vi "HW_QX - Parse Module Channel Parameters.vi"(8 "error in":errorcluster, 10 "sysModCFG[]":T5[](array[typedef]), 11 "AllDevRef[]":T3(array[cluster])) -> (0 "error out":errorcluster, 2 "InUsedDevRef[]":T3(array[cluster]), 3 "InUsedChan[]":T2)   [LabVIEW 2016]
uses:
  Ctrls/HardWare _ Channel Parameters.ctl
  Ctrls/HardWare _ Module Configuration.ctl
panel:
  out "AllModuPara[]":T4(array[cluster])
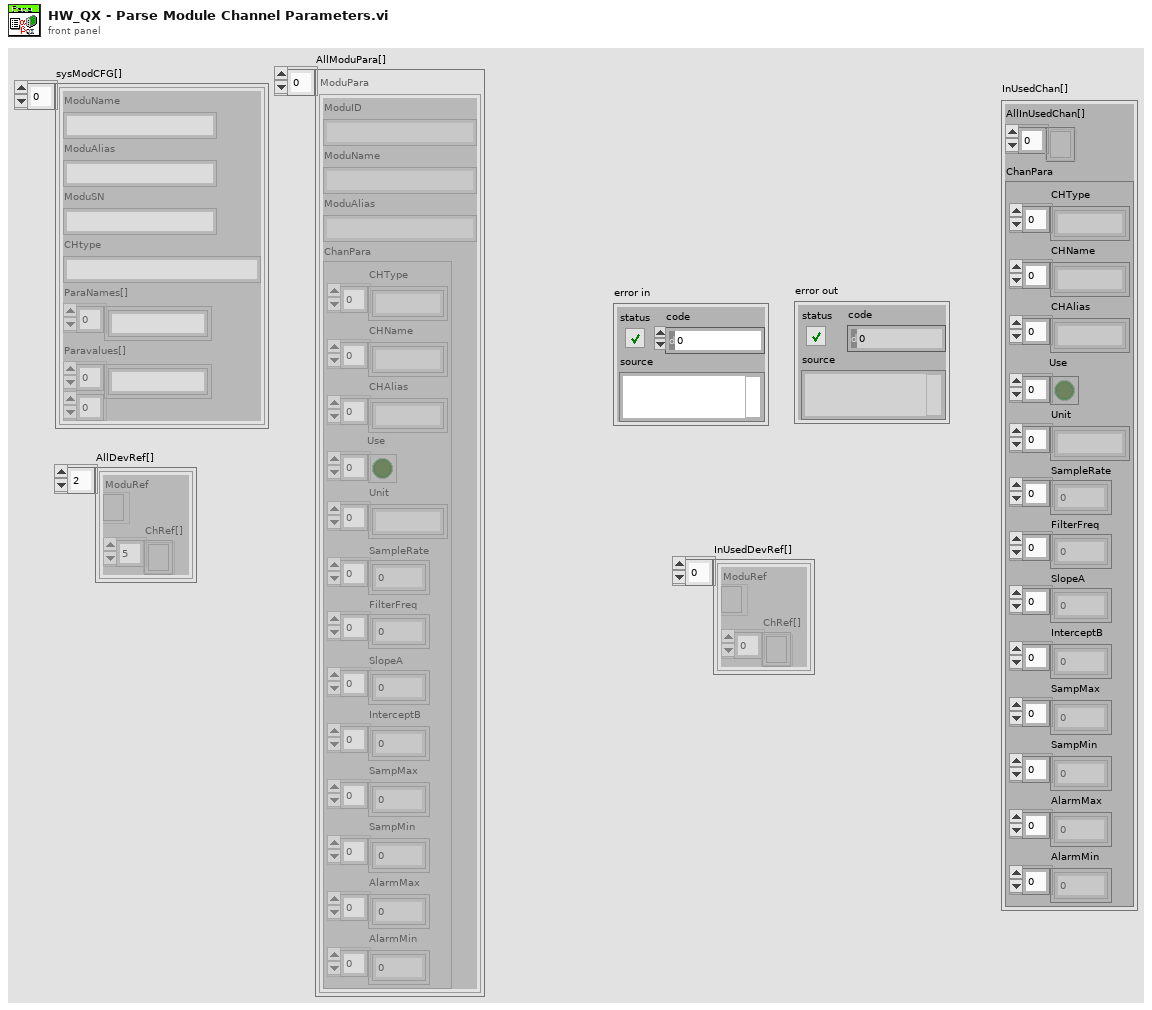
[diagram p1: front panel]
types:
  T1 = typedef "HardWare _ Channel Parameters.ctl" = cluster{"CHType":string[], "CHName":string[], "CHAlias":string[], "Use":bool[], "Unit":string[], "SampleRate":dbl[], "FilterFreq":dbl[], "SlopeA":dbl[], "InterceptB":dbl[], "SampMax":dbl[], "SampMin":dbl[], "AlarmMax":dbl[], "AlarmMin":dbl[]}
  T2 = cluster{"AllInUsedChan[]":refnum<k24>[], "ChanPara":T1}
  T3 = cluster{"ModuRef":refnum<k24>, "ChRef[]":refnum<k24>[]}[]
  T4 = cluster{"ModuID":string, "ModuName":string, "ModuAlias":string, "ChanPara":T1}[]
  T5 = typedef "HardWare _ Module Configuration.ctl" = cluster{"ModuName":string, "ModuAlias":string, "ModuSN":string, "CHtype":string, "ParaNames[]":string[], "Paravalues[]":string[][]}
  T6 = cluster{"ModuSN":string, "ModuName":string, "ModuAlias":string, "ChanPara":T1}
  T7 = cluster{string[], string[], string[], bool[], string[], dbl[], dbl[], dbl[], dbl[], dbl[], dbl[], dbl[], dbl[]}
  T8 = cluster{refnum<k24>[], cluster{string[], string[], string[], bool[], string[], dbl[], dbl[], dbl[], dbl[], dbl[], dbl[], dbl[], dbl[]}}
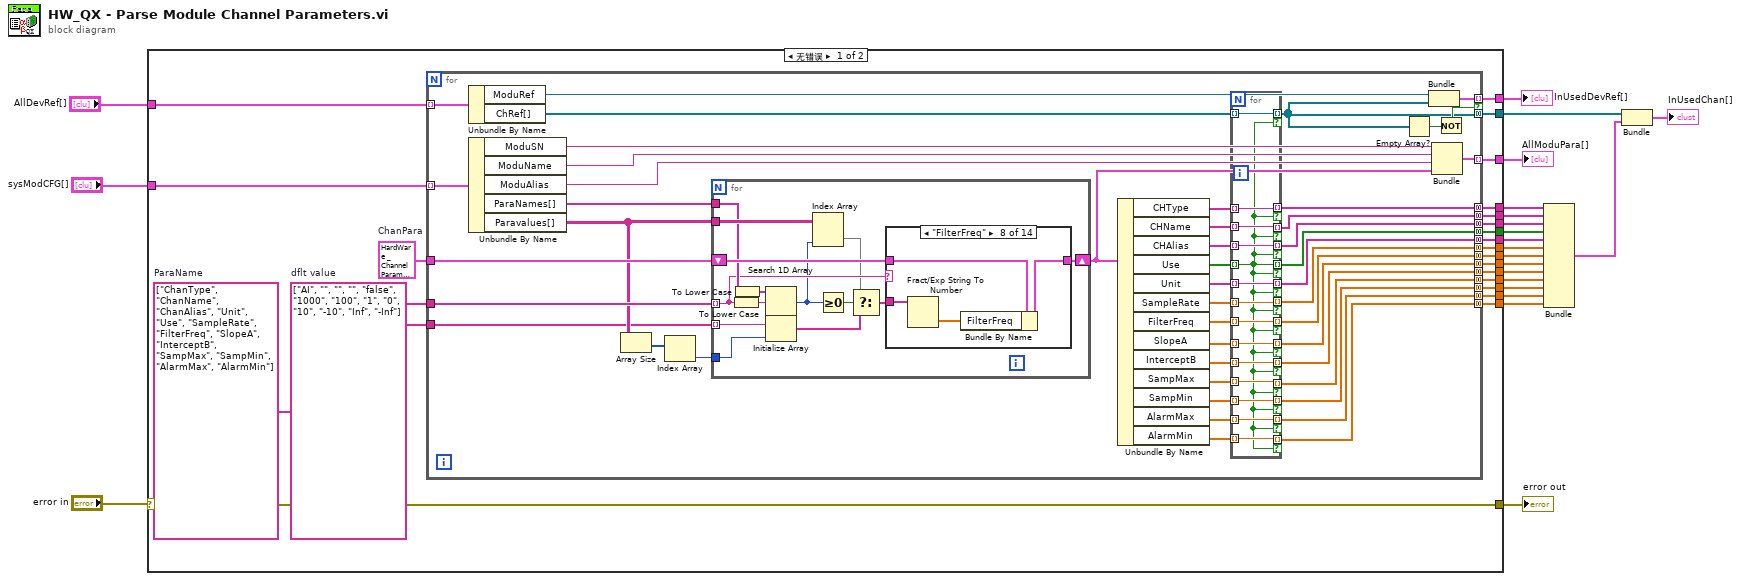
[diagram p0: block diagram]
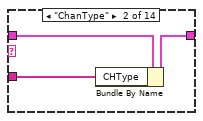
[diagram p3: hidden frame]
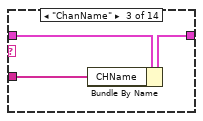
[diagram p4: hidden frame]
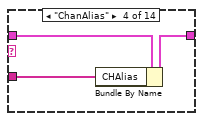
[diagram p5: hidden frame]
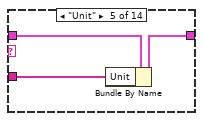
[diagram p6: hidden frame]
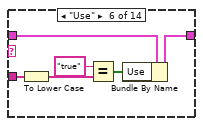
[diagram p7: hidden frame]
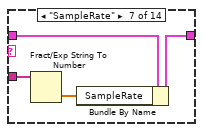
[diagram p8: hidden frame]
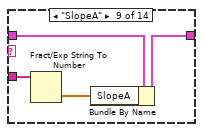
[diagram p9: hidden frame]
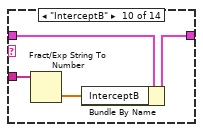
[diagram p10: hidden frame]
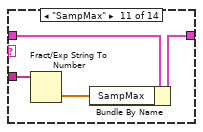
[diagram p11: hidden frame]
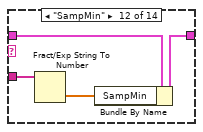
[diagram p12: hidden frame]
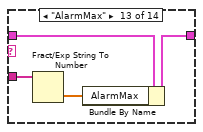
[diagram p13: hidden frame]
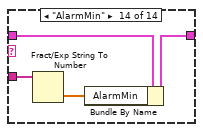
[diagram p14: hidden frame]
diagram:
  n1 = case shown="无错误" "error in" {
    selector: "error in" -> [w39 w170]
    tunnel: "sysModCFG[]" -> [w44 _]
    tunnel: [w40 _] -> w21
    tunnel: [w39 w170] -> w19
    tunnel: "AllDevRef[]" -> [w38 _]
    tunnel: [w37 _] -> w17
    tunnel: [w36 _] -> w2
    tunnel: [w35 _] -> w16
    tunnel: [w34 _] -> w15
    tunnel: [w33 _] -> w14
    tunnel: [w32 _] -> w13
    tunnel: [w31 _] -> w12
    tunnel: [w30 _] -> w11
    tunnel: [w29 _] -> w10
    tunnel: [w28 _] -> w9
    tunnel: [w27 _] -> w8
    tunnel: [w26 _] -> w7
    tunnel: [w25 _] -> w6
    tunnel: [w24 _] -> w5
    tunnel: [w23 _] -> w4
    frame No Error {
      w41 = string[] ["AI", "", "", "", "false", "1000", "100", "1", "0", "10", "-10", "Inf", "-Inf"]  # dflt value
      w42 = string[] ["ChanType", "ChanName", "ChanAlias", "Unit", "Use", "SampleRate", "FilterFreq", "SlopeA", "InterceptB", "SampMax", "SampMin", "AlarmMax", "AlarmMin"]  # ParaName
      w43 = T1 {"CHType"=[], "CHName"=[], "CHAlias"=[], "Use"=[], "Unit"=[], "SampleRate"=[], "FilterFreq"=[], "SlopeA"=[], "InterceptB"=[], "SampMax"=[], "SampMin"=[], "AlarmMax"=[], "AlarmMin"=[]}  # ChanPara
      n2 = for {
        tunnel: w44 -> [w90] mode=indexing
        tunnel: w43 -> [w88]
        tunnel: [w82] -> w40 mode=indexing
        tunnel: w42 -> [w87]
        tunnel: w41 -> [w83]
        tunnel: w38 -> [w63] mode=indexing
        tunnel: [w60] -> w37 mode=indexing if=w59
        tunnel: [w45] -> w36 mode=concatenating
        tunnel: [w58] -> w35 mode=concatenating
        tunnel: [w57] -> w34 mode=concatenating
        tunnel: [w56] -> w33 mode=concatenating
        tunnel: [w55] -> w32 mode=concatenating
        tunnel: [w54] -> w31 mode=concatenating
        tunnel: [w53] -> w30 mode=concatenating
        tunnel: [w52] -> w29 mode=concatenating
        tunnel: [w51] -> w28 mode=concatenating
        tunnel: [w50] -> w27 mode=concatenating
        tunnel: [w49] -> w26 mode=concatenating
        tunnel: [w48] -> w25 mode=concatenating
        tunnel: [w47] -> w24 mode=concatenating
        tunnel: [w46] -> w23 mode=concatenating
        n3 = Unbundle By Name(w63) -> ("ModuRef"=w61:refnum<k24>, "ChRef[]"=w62:refnum<k24>[])
        n4 = Unbundle By Name(w90) -> ("ModuSN"=w66:string, "ModuName"=w67:string, "ModuAlias"=w68:string, "ParaNames[]"=w89:string[], "Paravalues[]"=w86:string[][])
        n5 = Array Size(array=w86) -> (size(s)=w85:i32[])
        n6 = Index Array(array=w85) -> (element=w84:i32)  [unwired: 1 in]
        n7 = for {
          tunnel: w89 -> [w115]
          shift-right: [w116] -> w81
          shift-left: w88 -> [w118]
          tunnel: w86 -> [w117]
          tunnel: w87 -> [w114] mode=indexing
          tunnel: w84 -> [w111]
          tunnel: w83 -> [w110] mode=indexing
          n8 = To Lower Case(string=w114) -> (all lower case string=w105:string)
          n9 = To Lower Case(string=w115) -> (all lower case string=w106:string[])
          n10 = Search 1D Array(1D array=w106, element=w105) -> (index of element=w107:i32)  [unwired: 1 in]
          n11 = Initialize Array(w110, w111) -> (w109:string[])
          n12 = Index Array(array=w117, index (col)=w107) -> (element=w112:string[])  [unwired: 1 in]
          n13 = Greater Or Equal To 0?(x=w107) -> (x >= 0?=w113:bool)
          n14 = Select(t=w112, s=w113, f=w109) -> (s? t:f=w108:string[])
          n15 = case shown="\"FilterFreq\"" w114 {
            tunnel: w118 -> [w119 w122 w125 w128 w131 w137 w141 w145 w149 w153 w157 w161 w165 w169]
            tunnel: w108 -> [_ w120 w124 w127 w130 w136 w139 w143 w147 w151 w155 w159 w163 w167]
            tunnel: [w119 w121 w123 w126 w129 w135 w140 w144 w148 w152 w156 w160 w164 w168] -> w116
            frame Default {
            }
            frame "ChanType" {
              n16 = Bundle By Name(cluster=w122, "CHType"=w120) -> (w121:T1)
            }
            frame "ChanName" {
              n17 = Bundle By Name(cluster=w125, "CHName"=w124) -> (w123:T1)
            }
            frame "ChanAlias" {
              n18 = Bundle By Name(cluster=w128, "CHAlias"=w127) -> (w126:T1)
            }
            frame "Unit" {
              n19 = Bundle By Name(cluster=w131, "Unit"=w130) -> (w129:T1)
            }
            frame "Use" {
              n20 = To Lower Case(string=w136) -> (all lower case string=w134:string[])
              n21 = Equal?(x="true", y=w134) -> (x = y?=w133:bool[])
              n22 = Bundle By Name(cluster=w137, "Use"=w133) -> (w135:T1)
            }
            frame "SampleRate" {
              n23 = Fract/Exp String To Number(string=w139) -> (number=w138:dbl[])  [unwired: 3 in, 1 out]
              n24 = Bundle By Name(cluster=w141, "SampleRate"=w138) -> (w140:T1)
            }
            frame "FilterFreq" {
              n25 = Fract/Exp String To Number(string=w143) -> (number=w142:dbl[])  [unwired: 3 in, 1 out]
              n26 = Bundle By Name(cluster=w145, "FilterFreq"=w142) -> (w144:T1)
            }
            frame "SlopeA" {
              n27 = Fract/Exp String To Number(string=w147) -> (number=w146:dbl[])  [unwired: 3 in, 1 out]
              n28 = Bundle By Name(cluster=w149, "SlopeA"=w146) -> (w148:T1)
            }
            frame "InterceptB" {
              n29 = Fract/Exp String To Number(string=w151) -> (number=w150:dbl[])  [unwired: 3 in, 1 out]
              n30 = Bundle By Name(cluster=w153, "InterceptB"=w150) -> (w152:T1)
            }
            frame "SampMax" {
              n31 = Fract/Exp String To Number(string=w155) -> (number=w154:dbl[])  [unwired: 3 in, 1 out]
              n32 = Bundle By Name(cluster=w157, "SampMax"=w154) -> (w156:T1)
            }
            frame "SampMin" {
              n33 = Fract/Exp String To Number(string=w159) -> (number=w158:dbl[])  [unwired: 3 in, 1 out]
              n34 = Bundle By Name(cluster=w161, "SampMin"=w158) -> (w160:T1)
            }
            frame "AlarmMax" {
              n35 = Fract/Exp String To Number(string=w163) -> (number=w162:dbl[])  [unwired: 3 in, 1 out]
              n36 = Bundle By Name(cluster=w165, "AlarmMax"=w162) -> (w164:T1)
            }
            frame "AlarmMin" {
              n37 = Fract/Exp String To Number(string=w167) -> (number=w166:dbl[])  [unwired: 3 in, 1 out]
              n38 = Bundle By Name(cluster=w169, "AlarmMin"=w166) -> (w168:T1)
            }
          }
        }
        n39 = Unbundle By Name(w81) -> ("CHType"=w79:string[], "CHName"=w78:string[], "CHAlias"=w77:string[], "Use"=w80:bool[], "Unit"=w76:string[], "SampleRate"=w75:dbl[], "FilterFreq"=w64:dbl[], "SlopeA"=w74:dbl[], "InterceptB"=w73:dbl[], "SampMax"=w72:dbl[], "SampMin"=w71:dbl[], "AlarmMax"=w70:dbl[], "AlarmMin"=w69:dbl[])
        n40 = for {
          tunnel: w80 -> [w91] mode=indexing
          tunnel: w79 -> [w104] mode=indexing
          tunnel: w78 -> [w102] mode=indexing
          tunnel: w77 -> [w101] mode=indexing
          tunnel: w76 -> [w100] mode=indexing
          tunnel: w75 -> [w99] mode=indexing
          tunnel: w74 -> [w98] mode=indexing
          tunnel: w73 -> [w97] mode=indexing
          tunnel: w72 -> [w96] mode=indexing
          tunnel: w71 -> [w95] mode=indexing
          tunnel: w70 -> [w94] mode=indexing
          tunnel: w69 -> [w103] mode=indexing
          tunnel: [w104] -> w58 mode=indexing if=w91
          tunnel: [w103] -> w46 mode=indexing if=w91
          tunnel: [w102] -> w57 mode=indexing if=w91
          tunnel: [w101] -> w56 mode=indexing if=w91
          tunnel: [w100] -> w54 mode=indexing if=w91
          tunnel: [w99] -> w53 mode=indexing if=w91
          tunnel: [w98] -> w51 mode=indexing if=w91
          tunnel: [w97] -> w50 mode=indexing if=w91
          tunnel: [w96] -> w49 mode=indexing if=w91
          tunnel: [w95] -> w48 mode=indexing if=w91
          tunnel: [w94] -> w47 mode=indexing if=w91
          tunnel: [w91] -> w55 mode=indexing if=w91
          tunnel: w64 -> [w93] mode=indexing
          tunnel: [w93] -> w52 mode=indexing if=w91
          tunnel: w62 -> [w92] mode=indexing
          tunnel: [w92] -> w45 mode=indexing if=w91
        }
        n41 = Empty Array?(array=w45) -> (empty?=w65:bool)
        n42 = Bundle("ModuRef"=w61, w45) -> (w60:cluster{"ModuRef":refnum<k24>, refnum<k24>[]})  [unwired: 1 in]
        n43 = Bundle("ModuSN"=w66, "ModuName"=w67, "ModuAlias"=w68, "ChanPara"=w81) -> (w82:T6)  [unwired: 1 in]
        n44 = Not(x=w65) -> (.not. x?=w59:bool)
      }
    }
    frame Error {
    }
  }
  "AllModuPara[]" <- w21
  "error out" <- w19
  "InUsedDevRef[]" <- w17
  n45 = Bundle(w16, w15, w14, w13, w12, w11, w10, w9, w8, w7, w6, w5, w4) -> (w3:T7)  [unwired: 1 in]
  n46 = Bundle(w2, w3) -> (→"InUsedChan[]":T8)  [unwired: 1 in]
